vi "2D Helmholtz PDE Rendering (Rect Domain).vi"(0 "PDE in":refnum<class "NI_PDE.lvclass">, 5 "U(x, y)":dbl[][](array[numeric]), 11 "error in (no error)":errorcluster) -> (4 "PDE out":refnum<class "NI_PDE.lvclass">, 6 "PDE Plot":dbl[][](graph), 8 "X Scale":T1, 10 "Y Scale":T1, 15 "error out":errorcluster)   [LabVIEW 2020, in "NI_PDE.lvlib"]
doc: "Renders the solution of the partial differential equation. You must manually select the polymorphic instance to use."
uses:
  <vilib>/gmath/NI_PDE.lvlib
  <vilib>/gmath/pde.llb/PDEClass/NI_PDE.lvclass
  <vilib>/Utility/miscctls.llb/LVOffsetAndMultiplierTypeDef.ctl
  <vilib>/gmath/pde.llb/PDEClass/PDE_Helmholtz_2D/NI_PDE_Helmholtz_2D.lvclass
  e:/builds/penguin/labview/branches/2020/dev/dist/vi.lib/gmath/pde.llb/PDEClass/NI_PDE.lvclass
  <vilib>/gmath/pde.llb/DomainClass/Domain_Steady_2D_Rect/NI_Domain_Steady_2D_Rect.lvclass
  e:/builds/penguin/labview/branches/2020/dev/dist/vi.lib/gmath/pde.llb/DomainClass/NI_Domain.lvclass
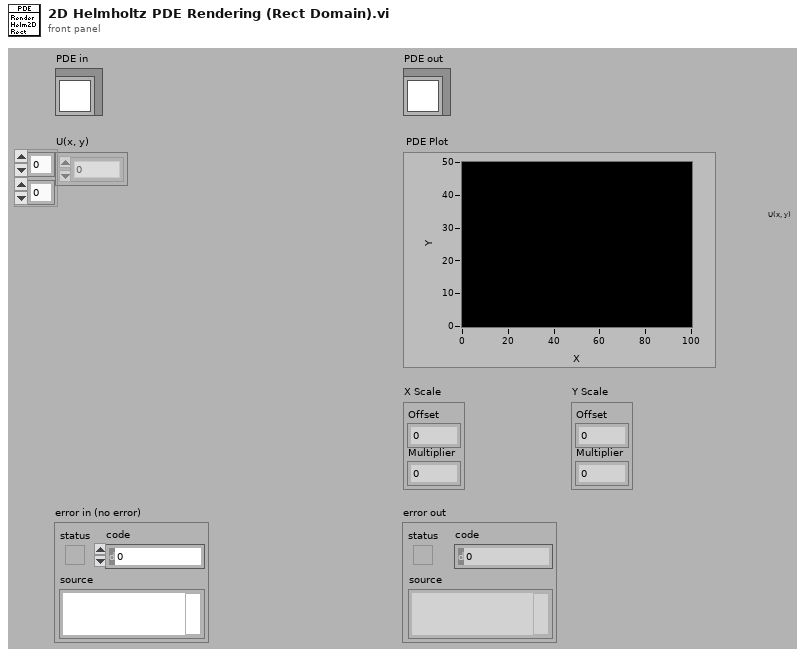
[diagram p1: front panel]
types:
  T1 = typedef "LVOffsetAndMultiplierTypeDef.ctl" = cluster{"Offset":dbl, "Multiplier":dbl}
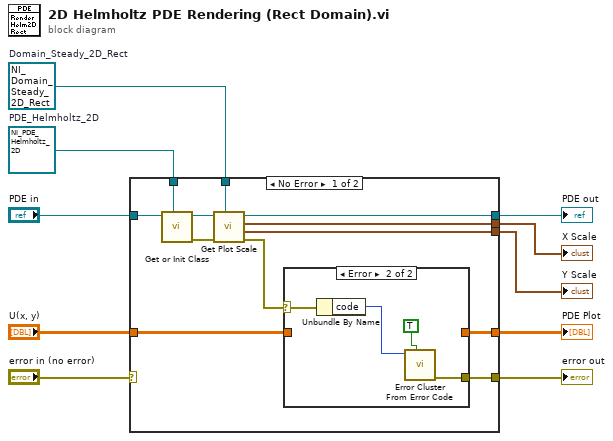
[diagram p0: block diagram]
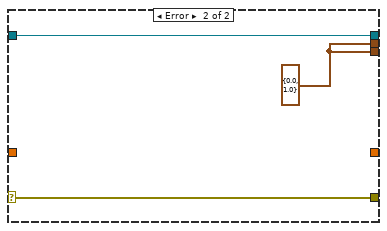
[diagram p3: hidden frame]
diagram:
  w3 = refnum<class "NI_Domain_Steady_2D_Rect.lvclass"> refnum  # Domain_Steady_2D_Rect
  w4 = refnum<class "NI_PDE_Helmholtz_2D.lvclass"> refnum  # PDE_Helmholtz_2D
  n1 = case shown="No Error" "error in (no error)" {
    selector: "error in (no error)" -> [_ w30]
    tunnel: "U(x, y)" -> [w22 _]
    tunnel: [w21 _] -> w9
    tunnel: [w16 w29] -> w8
    tunnel: "PDE in" -> [w20 w29]
    tunnel: [w19 w30] -> w6
    tunnel: w4 -> [w14 _]
    tunnel: w3 -> [w15 _]
    tunnel: [w12 w28] -> w1
    tunnel: [w11 w28] -> w2
    frame No Error {
      n2 = call <vilib>:"Get or Init Class.vi"("target PDE"=w14, "PDE in"=w20) -> ("error out"=w17:errorcluster, "PDE out"=w18:refnum<class "NI_PDE.lvclass">)  [unwired: 1 in, 7 out]
      n3 = call <vilib>:"Get Plot Scale.vi"("target Domain"=w15, "error in (no error)"=w17, "PDE in"=w18) -> ("error out"=w13:errorcluster, "Y Scale"=w12:T1, "X Scale"=w11:T1, "PDE out"=w16:refnum<class "NI_PDE.lvclass">)  [unwired: 5 out]
      n4 = case shown="Error" w13 {
        selector: w13 -> [_ w25]
        tunnel: w22 -> [w23 _]
        tunnel: [w23 _] -> w21
        tunnel: [_ w24] -> w19
        frame No Error {
        }
        frame Error {
          n5 = Unbundle By Name(w25) -> ("code"=w26:i32)
          n6 = call <vilib>:"Error Cluster From Error Code.vi"("show call chain? (False)"=TRUE, "error code (0)"=w26) -> ("error out"=w24:errorcluster)  [unwired: 1 in, 6 out]
        }
      }
    }
    frame Error {
      w28 = T1 {"Offset"=0.0, "Multiplier"=1.0} ("Offset and Multiplier")
    }
  }
  "PDE out" <- w8
  "error out" <- w6
  "PDE Plot" <- w9
  "X Scale" <- w2
  "Y Scale" <- w1
